vi "blink led.vi"() -> ()   [LabVIEW 2017]
panel:
  out "Boolean 4":bool
  out "Boolean 3":bool
  out "Boolean 2":bool
  out "Boolean":bool
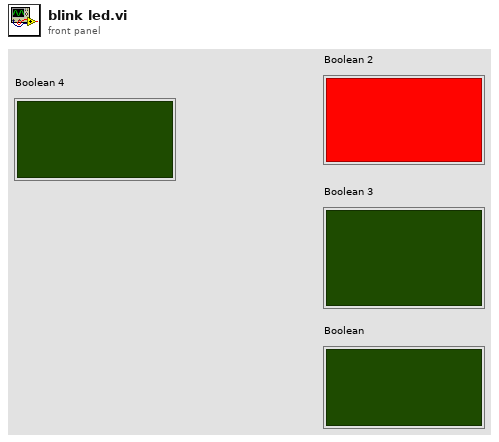
[diagram p1: front panel]
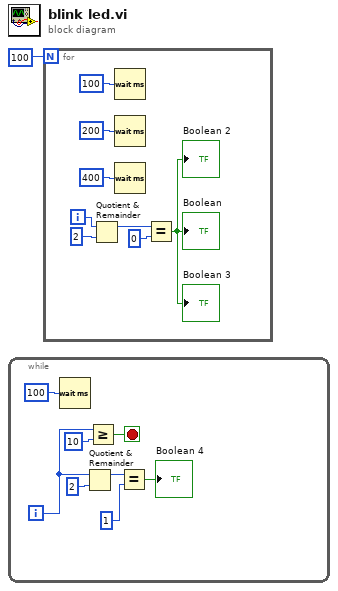
[diagram p0: block diagram]
diagram:
  n1 = while {
    i -> [w4]
    stop <- w2 stop-if-true
    n2 = Wait (ms)(milliseconds to wait=u32 100) -> ()  [unwired: 1 out]
    n3 = Quotient & Remainder(x=w4, y=2) -> (x-y*floor(x/y)=w8:i32)  [unwired: 1 out]
    n4 = Greater Or Equal?(x=w4, y=10) -> (x >= y?=w2:bool)
    n5 = Equal?(x=w8, y=1) -> (x = y?=→"Boolean 4":bool)
  }
  n6 = for {
    N: 100 -> [_]
    i -> [w17]
    n7 = Quotient & Remainder(x=w17, y=2) -> (x-y*floor(x/y)=w15:i32)  [unwired: 1 out]
    n8 = Wait (ms)(milliseconds to wait=u32 100) -> ()  [unwired: 1 out]
    n9 = Wait (ms)(milliseconds to wait=u32 200) -> ()  [unwired: 1 out]
    n10 = Wait (ms)(milliseconds to wait=u32 400) -> ()  [unwired: 1 out]
    n11 = Equal?(x=w15, y=0) -> (x = y?=→"Boolean" →"Boolean 2" →"Boolean 3":bool)
  }
